vi "test StatusAPI.vi"() -> ()   [LabVIEW 2017]
uses:
  user.lib/_NEVSTOP/Communicable State Machine(CSM)/_csmHelper/API/Create From VI Reference.vi
  user.lib/_NEVSTOP/Communicable State Machine(CSM)/_csmHelper/Properties/Read Status.vi
  user.lib/_NEVSTOP/Communicable State Machine(CSM)/_csmHelper/CSM-Helper.lvclass
panel:
  out "Array 3":cluster{"Status":string, "InState":string}[](array[cluster])
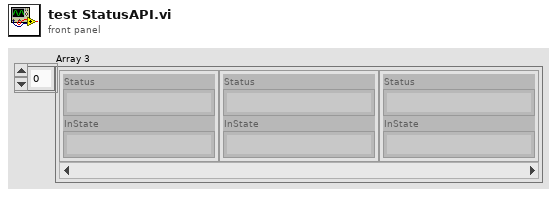
[diagram p1: front panel]
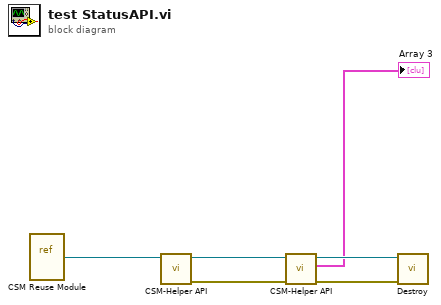
[diagram p0: block diagram]
diagram:
  n1 = vi-ref "CSM Reuse Module.vi"() -> (w3:refnum<vi>)
  n2 = call-poly "CSM-Helper API.vi"("VI"=w3) -> ("error out"=w4:errorcluster, "CSM-Helper.lvclass"=w5:refnum<class "CSM-Helper.lvclass">)  [unwired: 9 in]
  n3 = call-poly "CSM-Helper API.vi"("error in (no error)"=w4, "CSM-Helper in"=w5) -> ("error out"=w1:errorcluster, "Array 3"=→"Array 3":cluster{"Status":string, "InState":string}[], "CSM-Helper out"=w6:refnum<class "CSM-Helper.lvclass">)  [unwired: 7 in]
  n4 = call "Destroy.vi"("error in (no error)"=w1, "CSM-Helper in"=w6) -> ()  [unwired: 8 in, 2 out]
